vi "Main.vi"() -> ()   [LabVIEW 2013]
doc: "Use this template to build a simple state machine design pattern. Each state executes code and determines which state to transition to."
uses:
  controls/State.ctl
  controls/Data.ctl
  <vilib>/addons/zeromq/socket_type.ctl
  JSON RPC Request.ctl
  JSON RPC Response.ctl
  <userlib>/_OpenG.lib/file/file.llb/File Exists - Scalar__ogtk.vi
  <vilib>/addons/zeromq/zmq_context.lvclass
  <vilib>/addons/zeromq/zeromq.lvlib
  <vilib>/addons/zeromq/zmq_socket.lvclass
panel:
  in  "Output Directory":path
  out "State":T1
  in  "Capture":bool
  in  "Exit":bool
  # "These controls have associated \"Value Changed\" events configured in the Event Structure on the diagram.\n\nReplace them (and reconfigure the Event Structure) with the controls you need for your application."
  # "This template is for the Simple State Machine design pattern.\n\nSee the block diagram for more information on how to use this template."
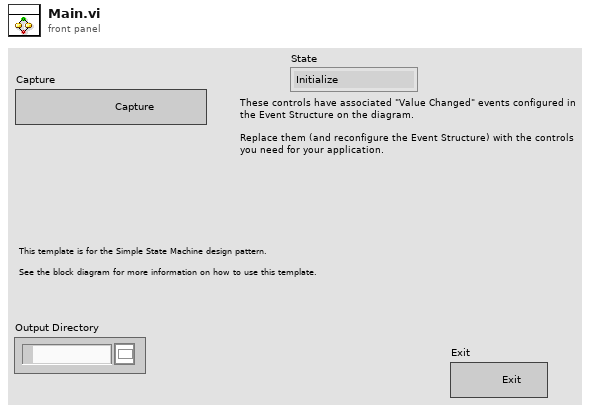
[diagram p1: front panel]
types:
  T1 = typedef "State.ctl" = enum16{"Initialize", "Wait for Event", "Capture", "Save Data", "Exit"}
  T2 = typedef "zeromq.lvlib/socket_type.ctl" = enum8{"ZMQ_PAIR", "ZMQ_PUB", "ZMQ_SUB", "ZMQ_REQ", "ZMQ_REP", "ZMQ_DEALER", "ZMQ_ROUTER", "ZMQ_PULL", "ZMQ_PUSH", "ZMQ_XPUB", "ZMQ_XSUB"}
  T3 = typedef "Data.ctl" = cluster{"Number of Samples":dbl, "Output Directory":path}
  T4 = enum8{"Enabled", "Disabled", "Disabled and Grayed Out"}
  T5 = typedef "JSON RPC Request.ctl" = cluster{"id":dbl, "method":string, "jsonrpc":string, "params":string[]}
  T6 = typedef "JSON RPC Response.ctl" = cluster{"id":dbl, "result":string, "jsonrpc":string}
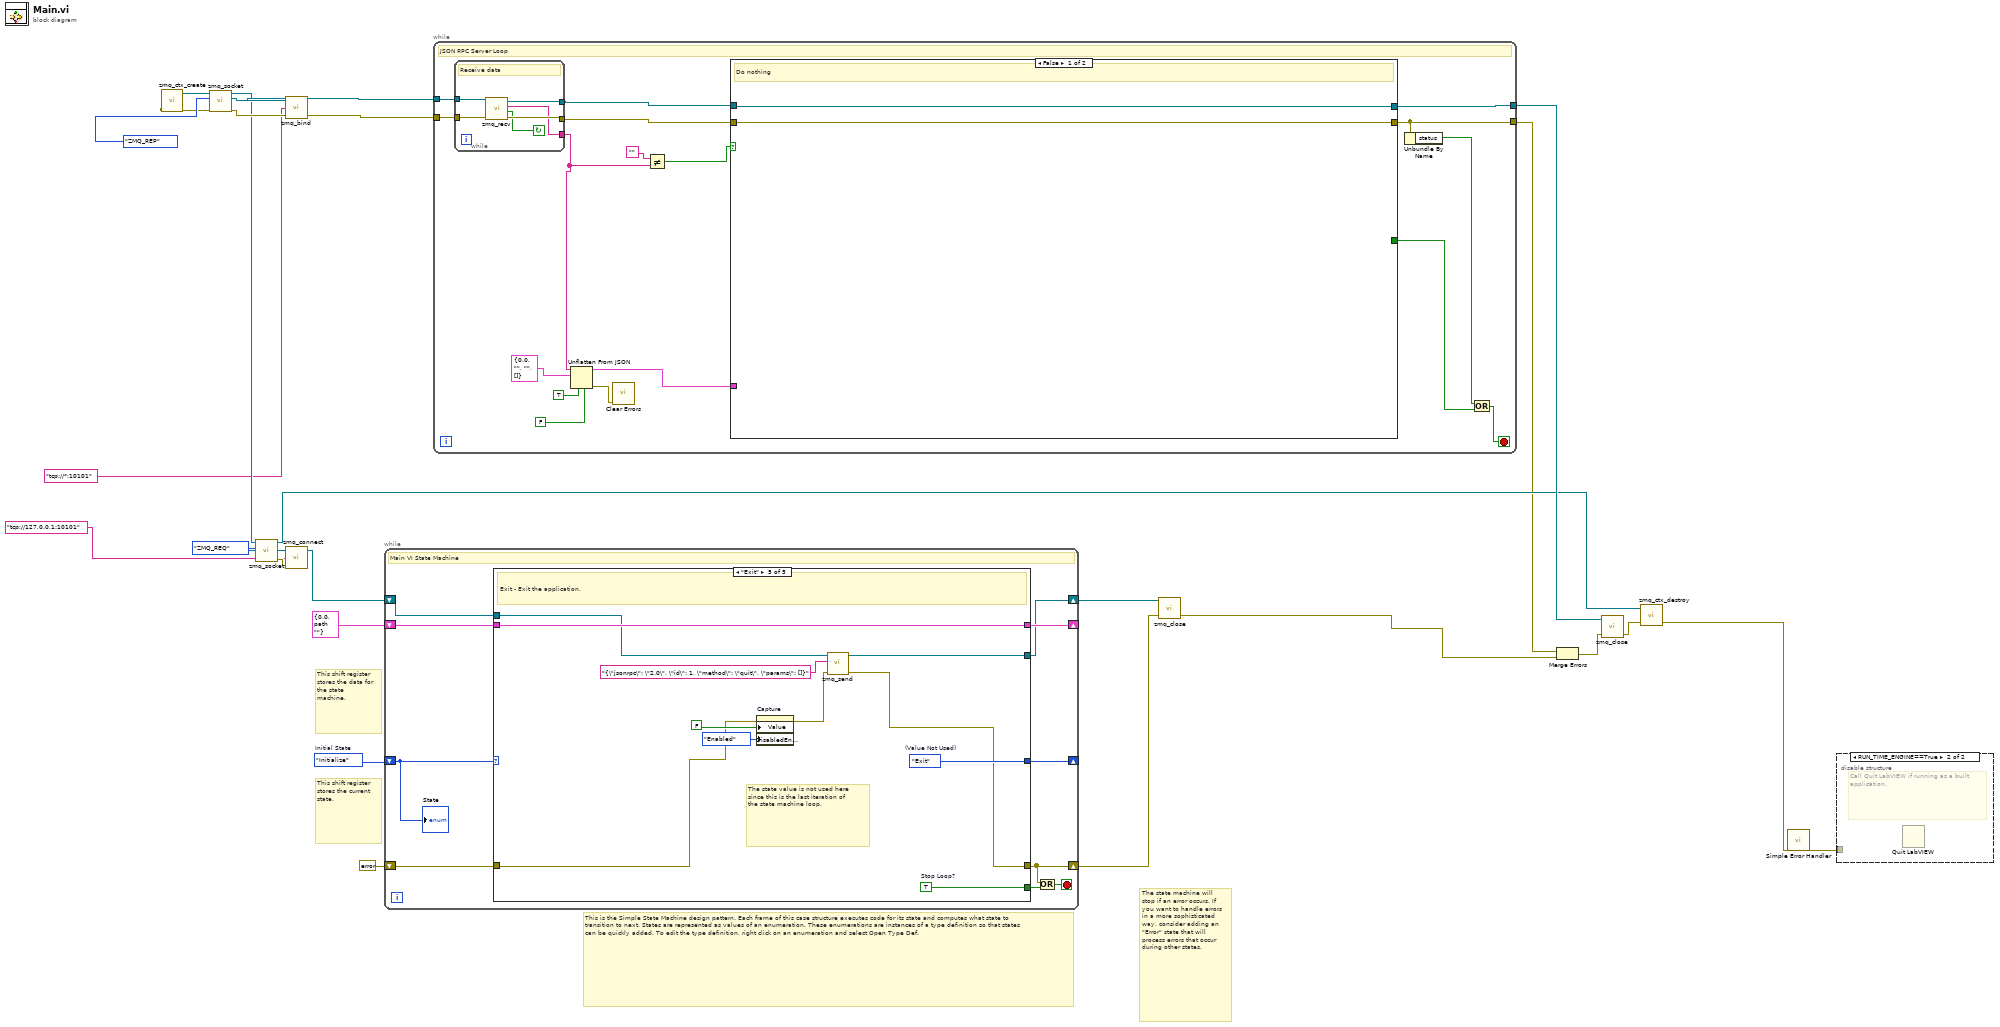
[diagram p0: block diagram]
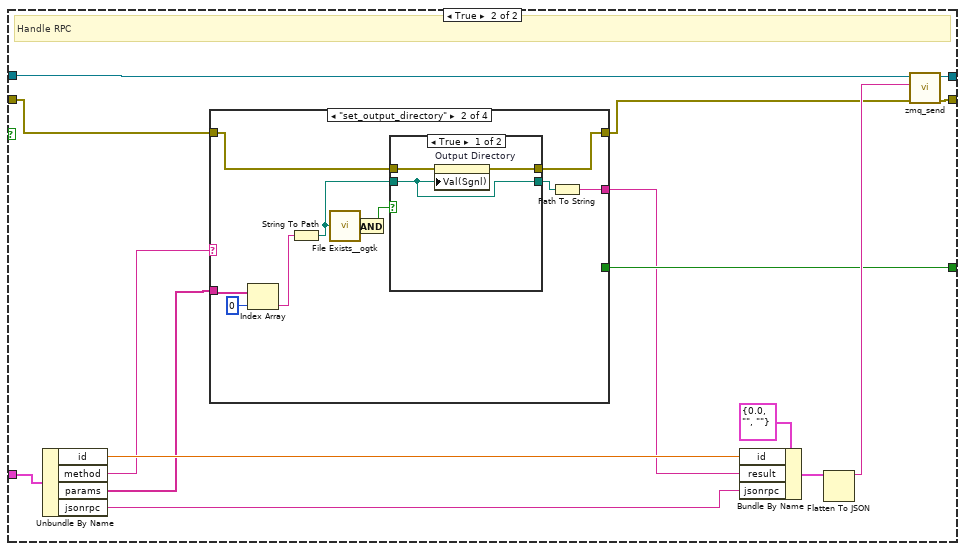
[diagram p2: hidden frame]
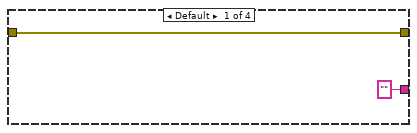
[diagram p3: hidden frame]
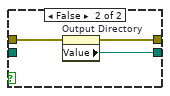
[diagram p4: hidden frame]
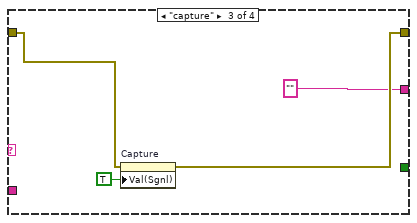
[diagram p5: hidden frame]
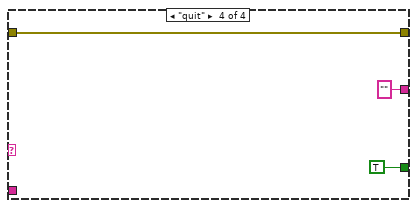
[diagram p6: hidden frame]
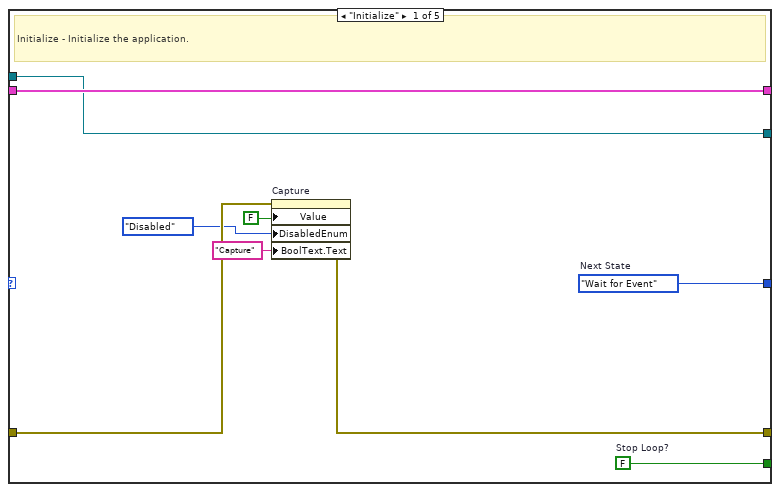
[diagram p8: hidden frame]
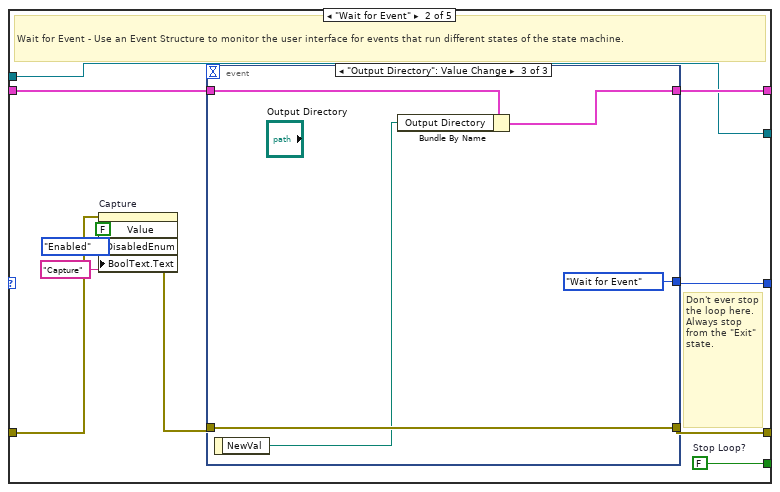
[diagram p9: hidden frame]
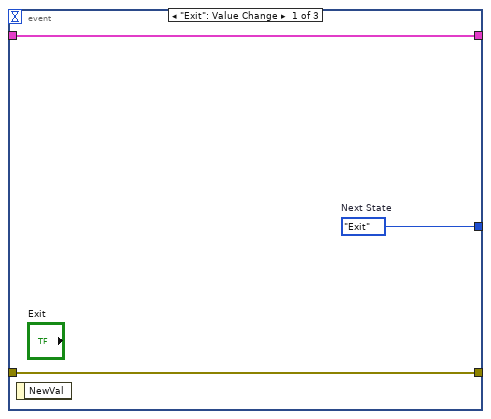
[diagram p10: hidden frame]
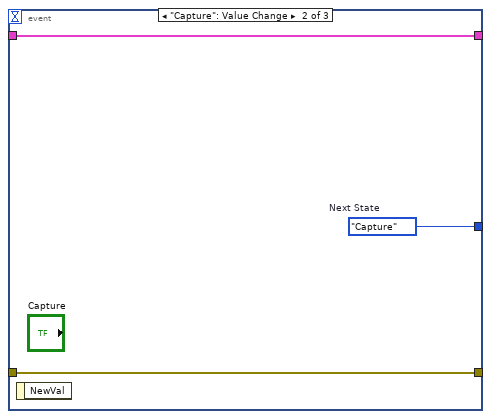
[diagram p11: hidden frame]
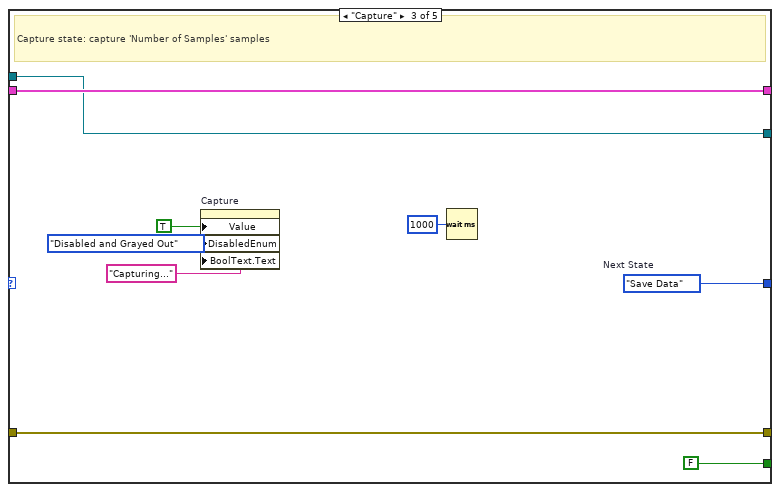
[diagram p12: hidden frame]
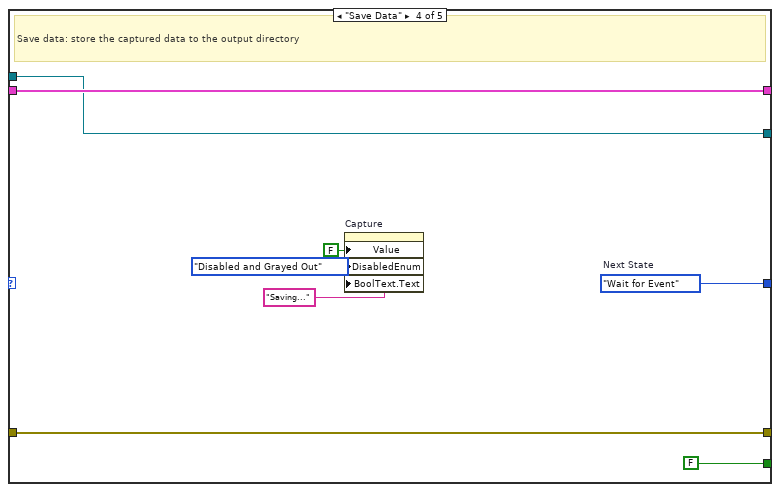
[diagram p13: hidden frame]
diagram:
  w27 = State."Initialize"  # Initial State
  # "The state machine will stop if an error occurs. If you want to handle errors in a more sophisticated way, consider adding an \"Error\" state that will process errors that occur during other states."
  # "This shift register stores the data for the state machine."
  # "This is the Simple State Machine design pattern. Each frame of this case structure executes code for its state and computes what state to transition to next. States are represented as values of an enumeration. These enumerations are instances of a type definition so that states can be quickly added. To edit the type definition, right click on an enumeration and select Open Type Def."
  # "This shift register stores the current state."
  n1 = call <vilib>:"zmq_ctx_create.vi"() -> ("error out"=w22:errorcluster, "context out"=w19:refnum<class "zmq_context.lvclass">)  [unwired: 4 in]
  n2 = call <vilib>:"zmq_socket.vi"("error in"=w22, "socket type"=socket_type."ZMQ_REP", "context in"=w19) -> ("error out"=w21:errorcluster, "socket out"=w20:refnum<class "zmq_socket.lvclass">, "context out"=w14:refnum<class "zmq_context.lvclass">)  [unwired: 2 in]
  n3 = call <vilib>:"zmq_socket.vi"("socket type"=socket_type."ZMQ_REQ", "context in"=w14) -> ("error out"=w9:errorcluster, "socket out"=w8:refnum<class "zmq_socket.lvclass">, "context out"=w12:refnum<class "zmq_context.lvclass">)  [unwired: 3 in]
  n4 = call <vilib>:"zmq_bind.vi"("error in"=w21, "endpoint"="tcp://*:10101", "socket in"=w20) -> ("error out"=w17:errorcluster, "socket out"=w18:refnum<class "zmq_socket.lvclass">)  [unwired: 1 in]
  n5 = call <vilib>:"zmq_connect.vi"("error in"=w9, "endpoint"="tcp://127.0.0.1:10101", "socket in"=w8) -> ("socket out"=w6:refnum<class "zmq_socket.lvclass">)  [unwired: 1 in, 1 out]
  n6 = while {
    shift-right: [w36] -> _
    shift-left: w27 -> [w37]
    shift-right: [w34] -> _
    shift-left: T3 {"Number of Samples"=0.0, "Output Directory"=path ""} ("Data") -> [w35]
    shift-right: [w30] -> w10
    shift-left: errorcluster {"status"=FALSE, "code"=0, "source"=""} ("error constant") -> [w33]
    shift-right: [w28] -> w11
    shift-left: w6 -> [w29]
    stop <- w31 stop-if-true
    # "Main VI State Machine"
    n7 = case shown="\"Exit\"" w37 {
      tunnel: [w46 w57 w77 w85 w96] -> w36
      tunnel: [w45 w56 FALSE ("Stop Loop?") FALSE ("Stop Loop?") w94] -> w32
      tunnel: w35 -> [w44 w55 w75 w83 w95]
      tunnel: [w44 w54 w75 w83 w95] -> w34
      tunnel: w33 -> [w41 w50 w74 w82 w88]
      tunnel: [w40 w53 w74 w82 w90] -> w30
      tunnel: w29 -> [w43 w52 w73 w81 w93]
      tunnel: [w43 w52 w73 w81 w91] -> w28
      frame "Initialize" {
        w45 = FALSE  # Stop Loop?
        w46 = State."Wait for Event"  # Next State
        # "Initialize - Initialize the application."
        n8 = property on="Capture" class="Bool (strict)"(error in=w41, "Value"=FALSE ("Capture"), "DisabledEnum"=T4."Disabled" ("Disabled"), "BoolText.Text"="Capture" ("Boolean Text.Text")) -> (error out=w40:errorcluster)  [unwired: 1 in, 1 out]
      }
      frame "Wait for Event" {
        w56 = FALSE  # Stop Loop?
        # "Don't ever stop the loop here. Always stop from the \"Exit\" state."
        # "Wait for Event - Use an Event Structure to monitor the user interface for events that run different states of the state machine."
        n9 = property on="Capture" class="Bool (strict)"(error in=w50, "Value"=FALSE ("Capture"), "DisabledEnum"=T4."Enabled" ("Disabled"), "BoolText.Text"="Capture" ("Boolean Text.Text")) -> (error out=w49:errorcluster)  [unwired: 1 in, 1 out]
        n10 = event shown="[2] \"Output Directory\": Value Change" {
          selector: _ -> [_ _ _]
          dyn-events: _ -> [_ _ _]
          timeout: _ -> [_ _ _]
          tunnel: [w60 w63 State."Wait for Event" ("Next State")] -> w57
          tunnel: w55 -> [w59 w61 w67]
          tunnel: [w59 w61 w66] -> w54
          tunnel: w49 -> [w58 w62 w68]
          tunnel: [w58 w62 w68] -> w53
          event "Exit": Value Change {
            w60 = State."Exit"  # Next State
            n11 = event-data() -> ()  [unwired: 1 in, 1 out]
          }
          event "Capture": Value Change {
            w63 = State."Capture"  # Next State
            n12 = event-data() -> ()  [unwired: 1 in, 1 out]
          }
          event "Output Directory": Value Change {
            n13 = event-data() -> ("NewVal"=w65:path)  [unwired: 1 in]
            n14 = Bundle By Name(cluster=w67, "Output Directory"=w65) -> (w66:T3)
          }
        }
      }
      frame "Capture" {
        w77 = State."Save Data"  # Next State
        # "Capture state: capture 'Number of Samples' samples"
        n15 = property on="Capture" class="Bool (strict)"("Value"=TRUE ("Capture"), "DisabledEnum"=T4."Disabled and Grayed Out" ("Disabled"), "BoolText.Text"="Capturing..." ("Boolean Text.Text")) -> ()  [unwired: 2 in, 2 out]
        n16 = Wait (ms)(milliseconds to wait=u32 1000) -> ()  [unwired: 1 out]
      }
      frame "Save Data" {
        w85 = State."Wait for Event"  # Next State
        # "Save data: store the captured data to the output directory"
        n17 = property on="Capture" class="Bool (strict)"("Value"=FALSE ("Capture"), "DisabledEnum"=T4."Disabled and Grayed Out" ("Disabled"), "BoolText.Text"="Saving..." ("Boolean Text.Text")) -> ()  [unwired: 2 in, 2 out]
      }
      frame "Exit" {
        w94 = TRUE  # Stop Loop?
        w96 = State."Exit"  # (Value Not Used)
        # "The state value is not used here since this is the last iteration of the state machine loop."
        # "Exit - Exit the application."
        n18 = property on="Capture" class="Bool (strict)"(error in=w88, "Value"=FALSE ("Capture"), "DisabledEnum"=T4."Enabled" ("Disabled")) -> (error out=w87:errorcluster)  [unwired: 1 in, 1 out]
        n19 = call <vilib>:"zmq_send.vi"("error in"=w87, "data"="{\"jsonrpc\": \"2.0\", \"id\": 1, \"method\": \"quit\", \"params\": []}", "socket in"=w93) -> ("error out"=w90:errorcluster, "socket out"=w91:refnum<class "zmq_socket.lvclass">)  [unwired: 4 in]
      }
    }
    n20 = Or(x=w30, y=w32) -> (x .or. y?=w31:bool)
    "State" <- w37
  }
  n21 = while {
    tunnel: [w104] -> w3
    tunnel: w18 -> [w112]
    tunnel: w17 -> [w111]
    tunnel: [w103] -> w15
    stop <- w99 stop-if-true
    # "JSON RPC Server Loop"
    n22 = while {
      tunnel: [w162] -> w110
      tunnel: [w161] -> w113
      tunnel: w112 -> [w159]
      tunnel: w111 -> [w158]
      tunnel: [w157] -> w107
      stop <- w160 continue-if-true
      # "Receive data"
      n23 = call <vilib>:"zmq_recv.vi"("error in"=w158, "socket in"=w159) -> ("error out"=w162:errorcluster, "more?"=w160:bool, "data"=w157:string, "socket out"=w161:refnum<class "zmq_socket.lvclass">)  [unwired: 3 in, 1 out]
    }
    n24 = Unflatten From JSON(JSON string=w107, type and defaults=T5 {"id"=0.0, "method"="", "jsonrpc"="", "params"=[]} ("JSON RPC Request"), default null elements? (F)=TRUE, strict validation? (F)=FALSE) -> (value=w109:T5, error out=w101:errorcluster)  [unwired: 3 in]
    n25 = call <vilib>:"Clear Errors.vi"("error in (no error)"=w101) -> ()  [unwired: 6 in, 1 out]
    n26 = Not Equal?(x="", y=w107) -> (x != y?=w105:bool)
    n27 = case shown="False" w105 {
      tunnel: w113 -> [w114 w130]
      tunnel: w110 -> [w115 w121]
      tunnel: w109 -> [_ w129]
      tunnel: [w115 w125] -> w104
      tunnel: [w114 w124] -> w103
      tunnel: [_ w117] -> w97
      frame False {
        # "Do nothing"
      }
      frame True {
        # "Handle RPC"
        n28 = Unbundle By Name(w129) -> ("id"=w127:dbl, "method"=w122:string, "params"=w118:string[], "jsonrpc"=w119:string)
        n29 = case shown="\"set_output_directory\"" w122 {
          tunnel: w121 -> [w132 w143 w153 w155]
          tunnel: [w132 w142 w152 w155] -> w120
          tunnel: w118 -> [_ w141 _ _]
          tunnel: [_ _ _ TRUE] -> w117
          tunnel: ["" w137 "" ""] -> w116
          frame Default {
          }
          frame "set_output_directory" {
            n30 = Index Array(array=w141, index=0) -> (element=w139:string)
            n31 = String To Path(string=w139) -> (path=w136:path)
            n32 = call-poly <userlib>:"File Exists__ogtk.vi"("file path"=w136) -> ("is directory"=w133:bool, "exists"=w134:bool)  [unwired: 6 in]
            n33 = And(x=w133, y=w134) -> (x .and. y?=w135:bool)
            n34 = case shown="True" w135 {
              tunnel: w143 -> [w146 w149]
              tunnel: [w145 w148] -> w142
              tunnel: w136 -> [w144 _]
              tunnel: [w144 w147] -> w138
              frame True {
                n35 = property on="Output Directory" class="Path"(error in=w146, "Val(Sgnl)"=w144) -> (error out=w145:errorcluster)  [unwired: 1 in, 1 out]
              }
              frame False {
                n36 = property on="Output Directory" class="Path"(error in=w149) -> (error out=w148:errorcluster, "Value"=w147:path)  [unwired: 1 in, 1 out]
              }
            }
            n37 = Path To String(path=w138) -> (string=w137:string)
          }
          frame "capture" {
            n38 = property on="Capture" class="Bool (strict)"(error in=w153, "Val(Sgnl)"=TRUE ("Value (Signaling)")) -> (error out=w152:errorcluster)  [unwired: 1 in, 1 out]
          }
          frame "quit" {
          }
        }
        n39 = Bundle By Name(cluster=T6 {"id"=0.0, "result"="", "jsonrpc"=""} ("JSON RPC Response"), "id"=w127, "result"=w116, "jsonrpc"=w119) -> (w128:T6)
        n40 = Flatten To JSON(anything=w128) -> (JSON string=w126:string)  [unwired: 2 in, 1 out]
        n41 = call <vilib>:"zmq_send.vi"("error in"=w120, "data"=w126, "socket in"=w130) -> ("error out"=w125:errorcluster, "socket out"=w124:refnum<class "zmq_socket.lvclass">)  [unwired: 4 in]
      }
    }
    n42 = Unbundle By Name(w104) -> ("status"=w98:bool)
    n43 = Or(x=w98, y=w97) -> (x .or. y?=w99:bool)
  }
  n44 = call <vilib>:"zmq_close.vi"("error in"=w10, "socket"=w11) -> ("error out"=w4:errorcluster)  [unwired: 3 in]
  n45 = Merge Errors(w3, w4) -> (w2:errorcluster)
  n46 = call <vilib>:"zmq_close.vi"("error in"=w2, "socket"=w15) -> ("error out"=w16:errorcluster)  [unwired: 3 in]
  n47 = call <vilib>:"zmq_ctx_destroy.vi"("error in"=w16, "context in"=w12) -> ("error out"=w1:errorcluster)  [unwired: 3 in]
  n48 = call <vilib>:"Simple Error Handler.vi"("error in (no error)"=w1) -> ("error out"=w24:errorcluster)  [unwired: 4 in, 4 out]
  n49 = disable-structure shown="RUN_TIME_ENGINE==True" {
    disable-tunnel: w24 -> [_ _]
    frame condition #0 (active) {
    }
    frame condition #1 {
      # "Call Quit LabVIEW if running as a built application."
      n50 = Quit LabVIEW() -> ()  [unwired: 1 in]
    }
  }
